vi "OSSP_Problem_Sort.vi"(8 "error in (no error)":errorcluster, 11 "OSSP_Problem.lvclass In":refnum<class "OSSP_Problem.lvclass">) -> (0 "error out":errorcluster, 3 "OSSP_Problem.lvclass Out":refnum<class "OSSP_Problem.lvclass">)   [LabVIEW 2013, in "OSSP_Problem.lvclass"]
uses:
  OSSP_Problem.lvclass
  OSSP_Problem.lvclass/OSSP_Problem.ctl
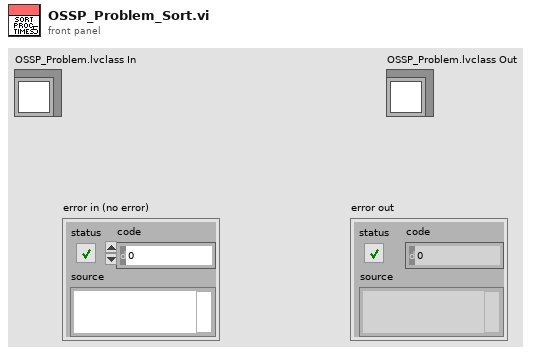
[diagram p1: front panel]
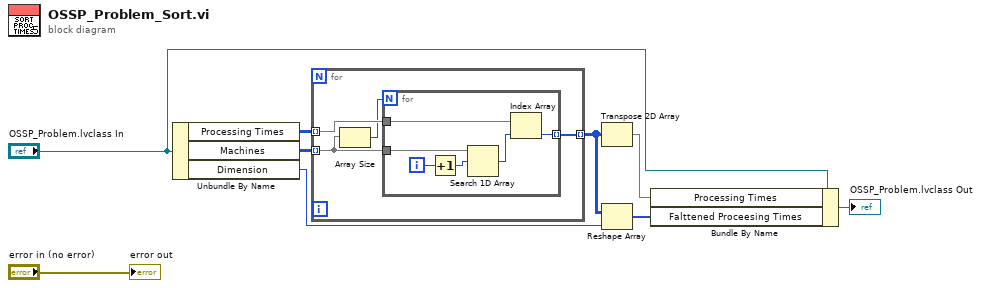
[diagram p0: block diagram]
diagram:
  n1 = Unbundle By Name("OSSP_Problem.lvclass In") -> ("Processing Times"=w9:u16[][], "Machines"=w8:u16[][], "Dimension"=w7:i32)
  n2 = for {
    tunnel: w9 -> [w13] mode=indexing
    tunnel: w8 -> [w11] mode=indexing
    tunnel: [w12] -> w2 mode=indexing
    n3 = Array Size(array=w11) -> (size(s)=w10:i32)
    n4 = for {
      N: w10 -> [_]
      tunnel: w11 -> [w14]
      tunnel: w13 -> [w15]
      tunnel: [w19] -> w12 mode=indexing
      i -> [w17]
      n5 = Increment(x=w17) -> (x+1=w18:i32)
      n6 = Search 1D Array(1D array=w14, element=w18) -> (index of element=w16:i32)  [unwired: 1 in]
      n7 = Index Array(array=w15, index=w16) -> (element=w19:u16)
    }
  }
  n8 = Transpose 2D Array(2D array=w2) -> (transposed array=w1:u16[][])
  n9 = Reshape Array(w2, w7) -> (w5:u16[])
  n10 = Bundle By Name(cluster="OSSP_Problem.lvclass In", "Processing Times"=w1, "Falttened Proceesing Times"=w5) -> (→"OSSP_Problem.lvclass Out":refnum<class "OSSP_Problem.lvclass">)
  "error out" <- "error in (no error)"
